vi "DLTS - timing calculation (emission rates) (SubVI).vi"(0 "Emission rates":dbl[unit][](array[numeric]) min=1.0 max=5000.0, 1 "Sampling rate":dbl(ring)=107142.859375 items=["13 kSa"=13392.857422, "27 kSa"=26785.714844, "54 kSa"=53571.429687, "107 kSa"=107142.859375], 2 "Averaging":i32=1, 3 "1st pulse duration":dbl[unit]=100.0 format="%#.1p", 4 "2nd Pulse duration":dbl[unit]=100.0 format="%#.1p", 5 "Acquisition delay":dbl[unit]=1.0 min=0.0 max=1.0 step=1e-06 format="%#_6p", 6 "2 pulse mode":bool) -> (14 "Number of samples":i32, 15 "Acquisition duration":dbl[unit], 16 "Pulse off time":dbl[unit])   [LabVIEW 2019]
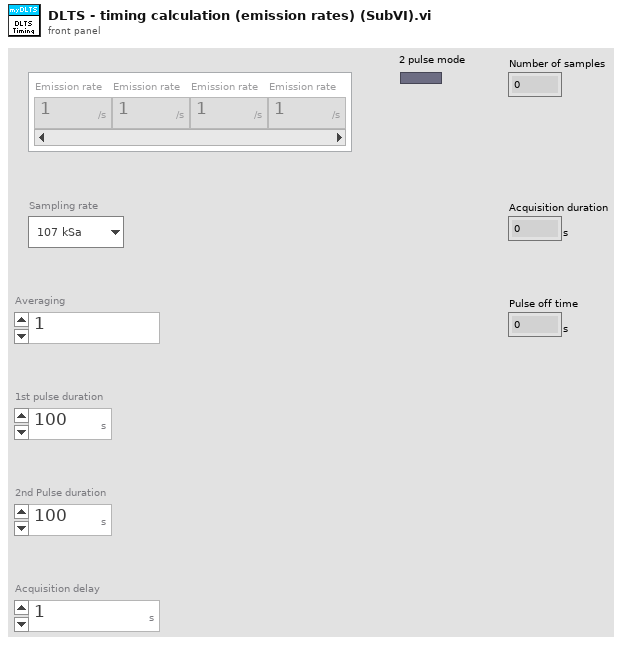
[diagram p1: front panel]
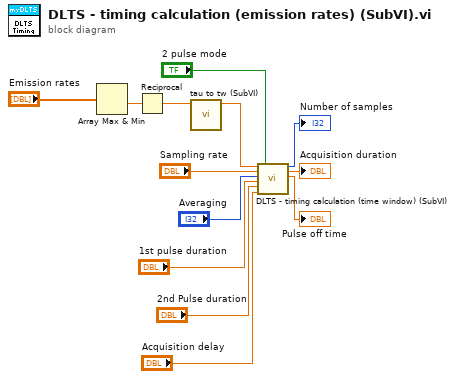
[diagram p0: block diagram]
diagram:
  n1 = Array Max & Min(array="Emission rates") -> (min value=w12:dbl[unit])  [unwired: 3 out]
  n2 = Reciprocal(x=w12) -> (1/x=w13:dbl[unit])
  n3 = call "tau to tw (SubVI).vi"("tau"=w13) -> ("t_w"=w10:dbl[unit])  [unwired: 9 in, 1 out]
  n4 = call "DLTS - timing calculation (time window) (SubVI).vi"("Time window"=w10, "Sampling rate"="Sampling rate", "Averaging"="Averaging", "1st pulse duration"="1st pulse duration", "2nd pulse duration"="2nd Pulse duration", "Acquisition delay"="Acquisition delay", "2 pulse mode"="2 pulse mode") -> ("Number of samples"=→"Number of samples":i32, "Acquisition duration"=→"Acquisition duration":dbl[unit], "Pulse off time"=→"Pulse off time":dbl[unit])  [unwired: 10 in]
